vi "FPGA_controller.vi"() -> ()   [LabVIEW 2017]
uses:
  <vilib>/rvi/Emulation/niFpgaGetClockAttributes.vi
  <vilib>/rvi/Emulation/niFpgaSctlEmulationGetInTimedLoop.vi
  <vilib>/rvi/Emulation/niFpgaEmulationReportErrorSimple.vi
  <vilib>/rvi/eio/common/nirviEmuTemplateMethod_errors.vi
  <vilib>/rvi/Emulation/niFpgaCriticalErrorInLSC.vi
  <vilib>/eio/EIONode/EIONode.xnode
panel:
  in  "m_first u2":fxp<+/-,64,32>=-0.8999999999068677 format="%#_42g"
  in  "m_first u1":fxp<+/-,64,32>=-0.8999999999068677 format="%#_42g"
  in  "Scale u2":fxp<+/-,64,42>=5.0 format="%#_35g"
  in  "Offset u2":fxp<+/-,64,41>=2.0 format="%#_36g"
  in  "Scale u1":fxp<+/-,64,42>=5.0 format="%#_35g"
  in  "Offset u1":fxp<+/-,64,41>=2.0 format="%#_36g"
  in  "eta u":fxp<+/-,64,32>=0.30000000004656613 format="%#_42g"
  in  "Scale x2":fxp<+/-,32,16>=10.0 format="%#_21g"
  in  "m_first x2":fxp<+/-,49,33> format="%#_26g"
  in  "Offset x2":fxp<+/-,48,32> format="%#_26g"
  in  "Offset x3":fxp<+/-,48,32>=5.0 format="%#_26g"
  in  "m_first x3":fxp<+/-,32,16>=-3.399993896484375 format="%#_21g"
  in  "Scale x3":fxp<+/-,32,16>=10.0 format="%#_21g"
  in  "1/eta x":fxp<+/-,32,16>=5.0 format="%#_21g"
  in  "m_first x1":fxp<+/-,49,33> format="%#_26g"
  in  "Offset x1":fxp<+/-,48,32> format="%#_26g"
  in  "Scale x1":fxp<+/-,32,16>=10.0 format="%#_21g"
  in  "stop":bool
  # "INPUTS CONVERSION"
  # "STATES CONVERSION"
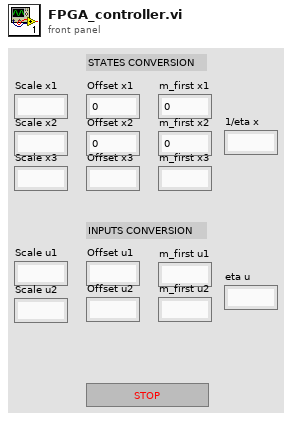
[diagram p1: front panel]
types:
  T1 = cluster{"Boolean array[0]":bool, "Boolean array[1]":bool, "Boolean array[2]":bool, "Boolean array[3]":bool, "Boolean array[4]":bool, "Boolean array[5]":bool, "Boolean array[6]":bool, "Boolean array[7]":bool, "Boolean array[8]":bool, "Boolean array[9]":bool, "Boolean array[10]":bool, "Boolean array[11]":bool, "Boolean array[12]":bool, "Boolean array[13]":bool, "Boolean array[14]":bool, "Boolean array[15]":bool, "Boolean array[16]":bool, "Boolean array[17]":bool}
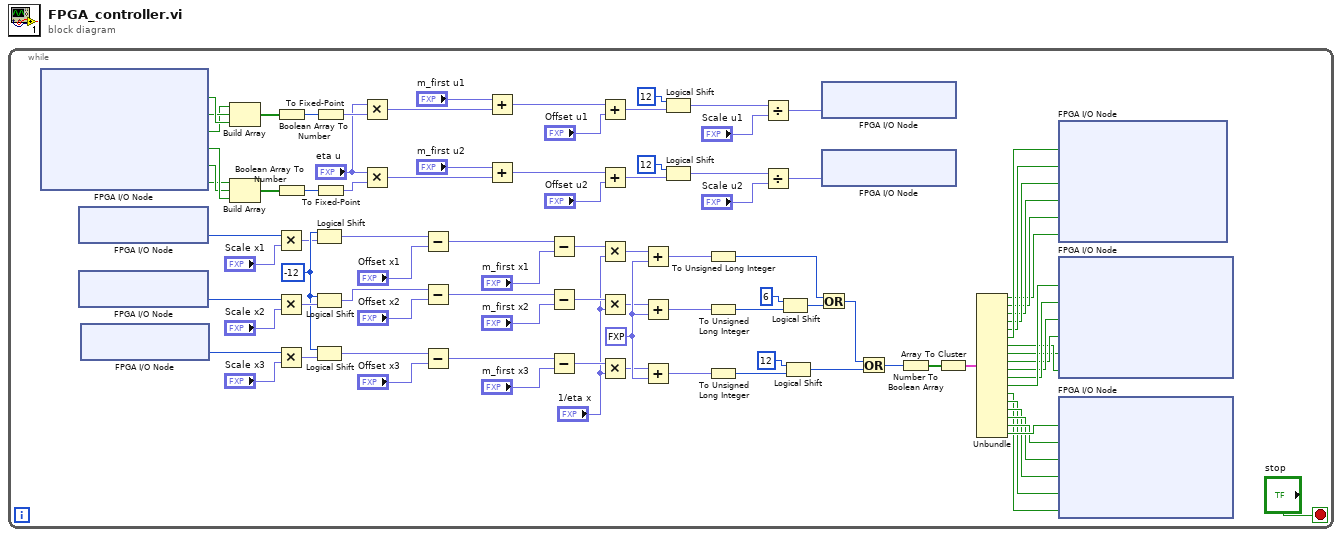
[diagram p0: block diagram]
diagram:
  n1 = while {
    stop <- "stop" stop-if-true
    w58 = fxp<+/-,64,32> 0.5 ("y")
    w51 = i16 -12 ("y")
    n2 = xnode "FPGA I/O Node"() -> ("Component-Level IP\\f0"=w24:bool, "Component-Level IP\\f1"=w23:bool, "Component-Level IP\\f2"=w22:bool, "Component-Level IP\\f3"=w21:bool, "Component-Level IP\\f4"=w20:bool, "Component-Level IP\\f5"=w19:bool)  [unwired: 6 in, 6 out]
    n3 = xnode "FPGA I/O Node"() -> ("ConnectorA/AI0"=w40:u16)  [unwired: 1 in, 1 out]
    n4 = xnode "FPGA I/O Node"() -> ("ConnectorA/AI1"=w50:u16)  [unwired: 1 in, 1 out]
    n5 = xnode "FPGA I/O Node"() -> ("ConnectorB/AI0"=w49:u16)  [unwired: 1 in, 1 out]
    n6 = Build Array(w22, w23, w24) -> (w92:bool[])
    n7 = Build Array(w19, w20, w21) -> (w80:bool[])
    n8 = Multiply(x=w40, y="Scale x1") -> (x*y=w39:fxp<+/-,48,32>)
    n9 = Multiply(x=w50, y="Scale x2") -> (x*y=w60:fxp<+/-,48,32>)
    n10 = Multiply(x=w49, y="Scale x3") -> (x*y=w46:fxp<+/-,48,32>)
    n11 = Boolean Array To Number(Boolean array=w92) -> (number=w88:u8)
    n12 = Boolean Array To Number(Boolean array=w80) -> (number=w77:u8)
    n13 = Logical Shift(y=w51, x=w39) -> (x << y=w35:fxp<+/-,48,32>)
    n14 = Logical Shift(y=w51, x=w60) -> (x << y=w29:fxp<+/-,48,32>)
    n15 = Logical Shift(y=w51, x=w46) -> (x << y=w45:fxp<+/-,48,32>)
    n16 = To Fixed-Point(number=w88) -> (fixed-point=w87:fxp<+,8,8>)  [unwired: 1 in]
    n17 = To Fixed-Point(number=w77) -> (fixed-point=w76:fxp<+,8,8>)  [unwired: 1 in]
    n18 = Multiply(x="eta u", y=w87) -> (x*y=w93:fxp<+/-,64,40>)
    n19 = Multiply(x="eta u", y=w76) -> (x*y=w81:fxp<+/-,64,40>)
    n20 = Subtract(x=w35, y="Offset x1") -> (x-y=w36:fxp<+/-,49,33>)
    n21 = Subtract(x=w29, y="Offset x2") -> (x-y=w31:fxp<+/-,49,33>)
    n22 = Subtract(x=w45, y="Offset x3") -> (x-y=w47:fxp<+/-,49,33>)
    n23 = Add(x="m_first u1", y=w93) -> (x+y=w91:fxp<+/-,64,41>)
    n24 = Add(x="m_first u2", y=w81) -> (x+y=w79:fxp<+/-,64,41>)
    n25 = Subtract(x=w36, y="m_first x1") -> (x-y=w38:fxp<+/-,50,34>)
    n26 = Subtract(x=w31, y="m_first x2") -> (x-y=w28:fxp<+/-,50,34>)
    n27 = Subtract(x=w47, y="m_first x3") -> (x-y=w55:fxp<+/-,50,34>)
    n28 = Add(x=w91, y="Offset u1") -> (x+y=w86:fxp<+/-,64,42>)
    n29 = Add(x=w79, y="Offset u2") -> (x+y=w75:fxp<+/-,64,42>)
    n30 = Multiply(x=w38, y="1/eta x") -> (x*y=w33:fxp<+/-,64,49>)
    n31 = Multiply(x=w28, y="1/eta x") -> (x*y=w26:fxp<+/-,64,49>)
    n32 = Multiply(x=w55, y="1/eta x") -> (x*y=w54:fxp<+/-,64,49>)
    n33 = Add(x=w33, y=w58) -> (x+y=w69:fxp<+/-,64,50>)
    n34 = Add(x=w26, y=w58) -> (x+y=w57:fxp<+/-,64,50>)
    n35 = Add(x=w54, y=w58) -> (x+y=w56:fxp<+/-,64,50>)
    n36 = Logical Shift(y=i16 12, x=w86) -> (x << y=w84:fxp<+/-,64,42>)
    n37 = Logical Shift(y=i16 12, x=w75) -> (x << y=w73:fxp<+/-,64,42>)
    n38 = To Unsigned Long Integer(number=w69) -> (unsigned 32bit integer=w65:u32)
    n39 = To Unsigned Long Integer(number=w57) -> (unsigned 32bit integer=w67:u32)
    n40 = To Unsigned Long Integer(number=w56) -> (unsigned 32bit integer=w63:u32)
    n41 = Divide(x=w84, y="Scale u1") -> (x/y=w82:fxp<+/-,64,65>)
    n42 = Divide(x=w73, y="Scale u2") -> (x/y=w72:fxp<+/-,64,65>)
    n43 = Logical Shift(y=6, x=w67) -> (x << y=w66:u32)
    n44 = Logical Shift(y=12, x=w63) -> (x << y=w62:u32)
    n45 = Or(x=w65, y=w66) -> (x .or. y?=w61:u32)
    n46 = xnode "FPGA I/O Node"("ConnectorB/AO0"=w82) -> ()  [unwired: 1 in, 1 out]
    n47 = xnode "FPGA I/O Node"("ConnectorB/AO1"=w72) -> ()  [unwired: 1 in, 1 out]
    n48 = Or(x=w61, y=w62) -> (x .or. y?=w44:u32)
    n49 = Number To Boolean Array(number=w44) -> (Boolean array=w70:bool[])
    n50 = Array To Cluster(array=w70) -> (cluster=w71:T1)
    n51 = Unbundle(w71) -> ("Boolean array[0]"=w13:bool, "Boolean array[1]"=w14:bool, "Boolean array[2]"=w15:bool, "Boolean array[3]"=w16:bool, "Boolean array[4]"=w17:bool, "Boolean array[5]"=w18:bool, "Boolean array[6]"=w8:bool, "Boolean array[7]"=w7:bool, "Boolean array[8]"=w9:bool, "Boolean array[9]"=w10:bool, "Boolean array[10]"=w11:bool, "Boolean array[11]"=w12:bool, "Boolean array[12]"=w1:bool, "Boolean array[13]"=w2:bool, "Boolean array[14]"=w3:bool, "Boolean array[15]"=w4:bool, "Boolean array[16]"=w5:bool, "Boolean array[17]"=w6:bool)
    n52 = xnode "FPGA I/O Node"("Component-Level IP\\x0"=w18, "Component-Level IP\\x1"=w17, "Component-Level IP\\x2"=w16, "Component-Level IP\\x3"=w15, "Component-Level IP\\x4"=w14, "Component-Level IP\\x5"=w13) -> ()  [unwired: 6 in, 6 out]
    n53 = xnode "FPGA I/O Node"("Component-Level IP\\x6"=w12, "Component-Level IP\\x7"=w11, "Component-Level IP\\x8"=w10, "Component-Level IP\\x9"=w9, "Component-Level IP\\x10"=w7, "Component-Level IP\\x11"=w8) -> ()  [unwired: 6 in, 6 out]
    n54 = xnode "FPGA I/O Node"("Component-Level IP\\x12"=w6, "Component-Level IP\\x13"=w5, "Component-Level IP\\x14"=w4, "Component-Level IP\\x15"=w3, "Component-Level IP\\x16"=w2, "Component-Level IP\\x17"=w1) -> ()  [unwired: 6 in, 6 out]
  }
